vi "KE622x -- Get Lin Log Sweep Params.vi"(0 "Resource In":refnum<visa-resource-name>, 1 "Check For SCPI Errors? (T)":bool=TRUE, 11 "error in (no error)":errorcluster) -> (4 "Resource Out (dupl)":refnum<visa-resource-name>, 8 "Lin Log Sweep Params":T1={"Sweep Type"=enum."Linear", "Source Delay (s)"=0.0, "Range Method"=enum."Fixed", "Num Sweeps"=enum."Sweep Count", "Sweep Count"=1, "Start Level (A)"=0.0, "Stop Level (A)"=0.1, "Step Level (A)"=0.01, "Num Steps"=11, "Abort On\nCompliance?"=FALSE} {"Num Steps" min=1 max=65535; "Step Level (A)" min=-0.105 max=0.105 format="%.4p"; "Stop Level (A)" min=-0.105 max=0.105 format="%.4p"; "Start Level (A)" min=-0.105 max=0.105 format="%.4p"; "Sweep Count" min=1 max=9999; "Source Delay (s)" min=0.001 max=1000.0 step=0.001 format="%.3f"}, 15 "error out":errorcluster)   [LabVIEW 2019, in "Keithley 622x.lvlib"]
doc: "Returns the parameters associated with a linear or log current sweep. The current set sweep type is indicated in 'Sweep Type'. Note that 'Step Level (A)' only applies to linear sweeps."
uses:
  Keithley 622x.lvlib
  Typedefs/KE622x -- Lin Log Sweep Params.ctl
  Typedefs/KE622x -- Source Delay.ctl
  Typedefs/KE622x -- Current Level.ctl
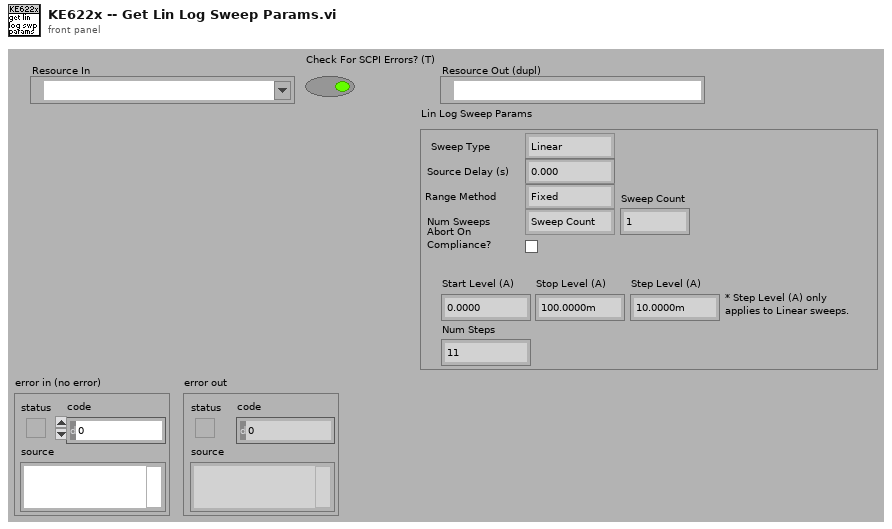
[diagram p1: front panel]
types:
  T1 = typedef "Keithley 622x.lvlib/KE622x -- Lin Log Sweep Params.ctl" = cluster{"Sweep Type":enum16{"Linear", "Log", "List"}, "Source Delay (s)":T2, "Range Method":enum16{"Auto", "Best", "Fixed"}, "Num Sweeps":enum16{"Sweep Count", "Infinite"}, "Sweep Count":u32, "Start Level (A)":T3, "Stop Level (A)":T3, "Step Level (A)":T3, "Num Steps":u32, "Abort On\nCompliance?":bool}
  T2 = typedef "Keithley 622x.lvlib/KE622x -- Source Delay.ctl" = dbl
  T3 = typedef "Keithley 622x.lvlib/KE622x -- Current Level.ctl" = dbl
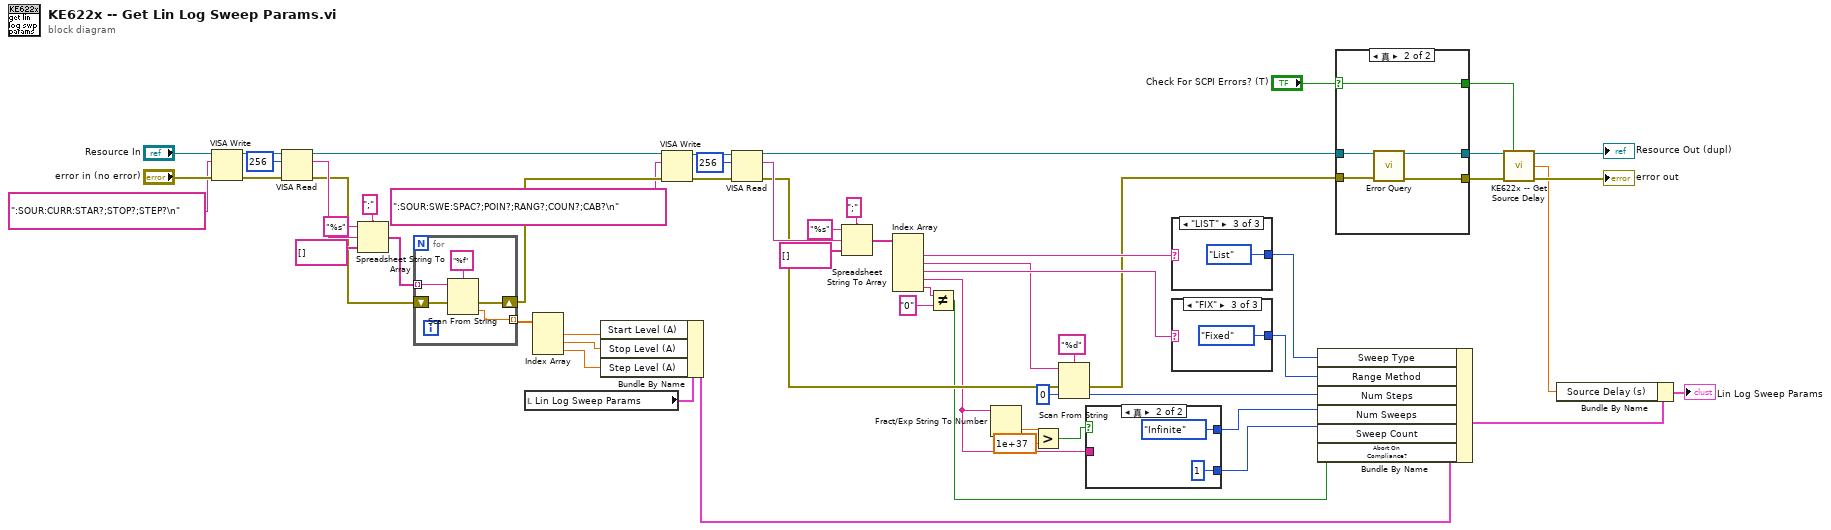
[diagram p0: block diagram]
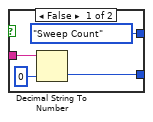
[diagram p2: hidden frame]
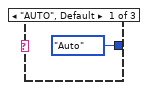
[diagram p3: hidden frame]
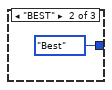
[diagram p4: hidden frame]
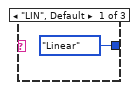
[diagram p5: hidden frame]
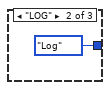
[diagram p6: hidden frame]
diagram:
  n1 = VISA Write(VISA resource name="Resource In", write buffer=":SOUR:CURR:STAR?;STOP?;STEP?\n" ("format string"), error in (no error)="error in (no error)") -> (VISA resource name out=w54:refnum<visa-resource-name>, error out=w53:errorcluster)  [unwired: 1 out]
  n2 = VISA Read(VISA resource name=w54, byte count=u32 256, error in (no error)=w53) -> (VISA resource name out=w37:refnum<visa-resource-name>, read buffer=w51:string, error out=w46:errorcluster)  [unwired: 1 out]
  n3 = Spreadsheet String To Array(delimiter (Tab)=";", format string="%s", spreadsheet string=w51, array type (2D Dbl)=string[] []) -> (array=w45:string[])
  n4 = for {
    shift-right: [w60] -> w36
    shift-left: w46 -> [w63]
    tunnel: w45 -> [w62] mode=indexing
    tunnel: [w59] -> w44 mode=indexing
    n5 = Scan From String(format string="%f", input string=w62, error in=w63) -> (error out=w60:errorcluster, output 1=w59:dbl)  [unwired: 2 in, 2 out]
  }
  n6 = local read "Lin Log Sweep Params"() -> (w47:T1)
  n7 = Index Array(array=w44) -> (element #1=w43:dbl, element #2=w42:dbl, element #3=w41:dbl)  [unwired: 3 in]
  n8 = Bundle By Name(cluster=w47, "Start Level (A)"=w43, "Stop Level (A)"=w42, "Step Level (A)"=w41) -> (w27:T1)
  n9 = VISA Write(VISA resource name=w37, write buffer=":SOUR:SWE:SPAC?;POIN?;RANG?;COUN?;CAB?\n", error in (no error)=w36) -> (VISA resource name out=w40:refnum<visa-resource-name>, error out=w39:errorcluster)  [unwired: 1 out]
  n10 = VISA Read(VISA resource name=w40, byte count=u32 256, error in (no error)=w39) -> (VISA resource name out=w14:refnum<visa-resource-name>, read buffer=w31:string, error out=w29:errorcluster)  [unwired: 1 out]
  n11 = Spreadsheet String To Array(delimiter (Tab)=";", format string="%s", spreadsheet string=w31, array type (2D Dbl)=string[] []) -> (array=w30:string[])
  n12 = Index Array(array=w30) -> (element #1=w28:string, element #2=w21:string, element #3=w25:string, element #4=w7:string, element #5=w3:string)  [unwired: 5 in]
  n13 = Not Equal?(x=w3, y="0") -> (x != y?=w1:bool)
  n14 = Fract/Exp String To Number(string=w7) -> (number=w6:dbl)  [unwired: 3 in, 1 out]
  n15 = Greater?(x=w6, y=1e+37) -> (0:w4:bool)
  n16 = Scan From String(format string="%d", input string=w21, error in=w29, default 1=u32 0 ("default value 1")) -> (error out=w15:errorcluster, output 1=w20:u32)  [unwired: 1 in, 2 out]
  n17 = case shown="真" w4 {
    tunnel: [enum16{"Sweep Count", "Infinite"}."Sweep Count" ("Num Sweeps") enum16{"Sweep Count", "Infinite"}."Infinite" ("Num Sweeps")] -> w19
    tunnel: w7 -> [w66 _]
    tunnel: [w64 u32 1] -> w18
    frame False {
      n18 = Decimal String To Number(string=w66, default (0L)=u32 0 ("default (0 I32)")) -> (number=w64:u32)  [unwired: 1 in, 1 out]
    }
    frame True {
    }
  }
  n19 = case shown="\"LIST\"" w28 {
    tunnel: [enum16{"Linear", "Log", "List"}."Linear" ("Sweep Type") enum16{"Linear", "Log", "List"}."Log" ("Sweep Type") enum16{"Linear", "Log", "List"}."List" ("Sweep Type")] -> w26
    frame "LIN", Default {
    }
    frame "LOG" {
    }
    frame "LIST" {
    }
  }
  n20 = case shown="\"FIX\"" w25 {
    tunnel: [enum16{"Auto", "Best", "Fixed"}."Auto" ("Range Method") enum16{"Auto", "Best", "Fixed"}."Best" ("Range Method") enum16{"Auto", "Best", "Fixed"}."Fixed" ("Range Method")] -> w24
    frame "AUTO", Default {
    }
    frame "BEST" {
    }
    frame "FIX" {
    }
  }
  n21 = Bundle By Name(cluster=w27, "Sweep Type"=w26, "Range Method"=w24, "Num Steps"=w20, "Num Sweeps"=w19, "Sweep Count"=w18, "Abort On\nCompliance?"=w1) -> (w17:T1)
  n22 = case shown="真" "Check For SCPI Errors? (T)" {
    selector: "Check For SCPI Errors? (T)" -> [w76 w81]
    tunnel: w14 -> [w78 w83]
    tunnel: [w77 w79] -> w11
    tunnel: [w78 w82] -> w13
    tunnel: w15 -> [w77 w80]
    tunnel: [w76 w81] -> w12
    frame False {
    }
    frame True {
      n23 = call "Error Query.vi"("VISA Resource In"=w83, "error in (no error)"=w80) -> ("VISA Resource Out (dupl)"=w82:refnum<visa-resource-name>, "error out"=w79:errorcluster)  [unwired: 10 in, 2 out]
    }
  }
  n24 = call "KE622x -- Get Source Delay.vi"("Resource In"=w13, "Check For SCPI Errors? (T)"=w12, "error in (no error)"=w11) -> ("Resource Out (dupl)"=→"Resource Out (dupl)":refnum<visa-resource-name>, "Source Delay (s)"=w8:T2, "error out"=→"error out":errorcluster)  [unwired: 10 in]
  n25 = Bundle By Name(cluster=w17, "Source Delay (s)"=w8) -> (→"Lin Log Sweep Params":T1)
